vi "Launch Nested Actors.vi"(8 "error in (no error)":errorcluster, 11 "Preparation Line in":refnum<class "Preparation Line.lvclass">) -> (0 "error out":errorcluster, 3 "Preparation Line out":refnum<class "Preparation Line.lvclass">)   [LabVIEW 2015, in "cRIO-Carbondioxide.lvlib" / "CO2-Actor.lvlib" / "Preparation Line.lvclass"]
uses:
  Preparation Line.lvclass
  <vilib>/ActorFramework/Actor/Actor.lvclass
  Valve/Action.ctl
  Preparation Line.lvclass/Preparation Line.ctl
  CO2 Actor/CO2 Actor.lvclass
  Valve/Valve.lvclass
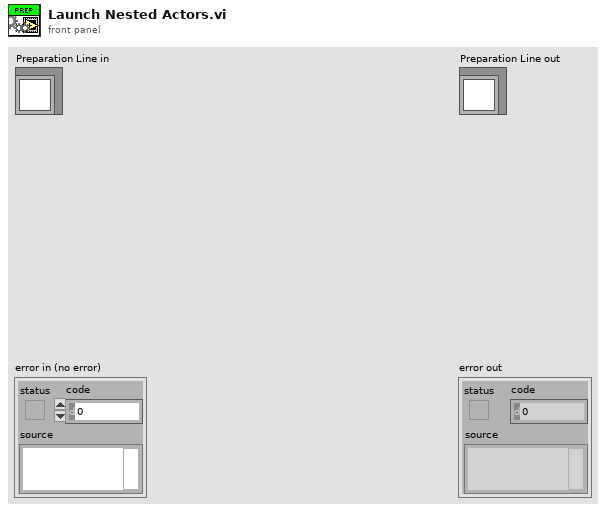
[diagram p1: front panel]
types:
  T1 = typedef "Action.ctl" = enum16{"Open", "Close", "None"}
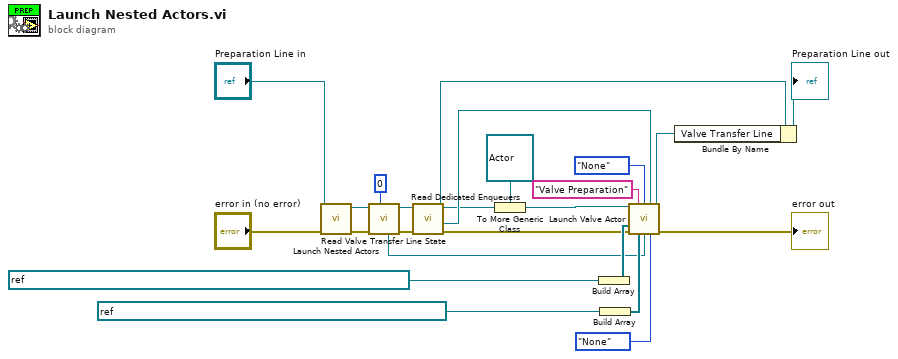
[diagram p0: block diagram]
diagram:
  n1 = call-parent "Launch Nested Actors.vi"("error in (no error)"="error in (no error)", "CO2 Actor in"="Preparation Line in") -> ("error out"=w8:errorcluster, "CO2 Actor out"=w5:refnum<class "Preparation Line.lvclass">)  [unwired: 8 in]
  n2 = call "Read Valve Transfer Line State.vi"("timeout in ms (-1)"=0, "error in (no error)"=w8, "Preparation Line in"=w5) -> ("error out"=w7:errorcluster, "Preparation Line out"=w6:refnum<class "Preparation Line.lvclass">, "Valve Prep Line StateQ"=w3:refnum<queue>)  [unwired: 5 in, 1 out]
  n3 = call "Read Dedicated Enqueuers.vi"("error in (no error)"=w7, "CO2 Actor in"=w6) -> ("error out"=w10:errorcluster, "DedicatedEnQrs"=w9:refnum<queue>, "CO2 Actor out"=w4:refnum<class "Preparation Line.lvclass">)  [unwired: 6 in, 1 out]
  n4 = To More Generic Class(target class=refnum<class "Actor.lvclass"> refnum ("Caller Actor in"), reference=w4) -> (generic class reference=w17:refnum<class "Actor.lvclass">)
  n5 = Build Array(refnum<k21> "ni.var.psp://crio-carbondioxide/AMS Gas SHV/Valves/Prep Line Valve 0" ("SHV")) -> (w11:refnum<k21>[])
  n6 = Build Array(refnum<k21> "ni.var.io://crio-carbondioxide/Mod2/Prep Line Valve 0 DV300" ("SHV")) -> (w19:refnum<k21>[])
  n7 = call "Launch Valve Actor.vi"("Caller Actor in"=w17, "Name"="Valve Preparation", "Start Action (Open)"=Action."None", "DedicatedEnQrs"=w9, "SHV Aliases"=w11, "error in (no error)"=w10, "SHV"=w19, "StateQ"=w3, "Stop Action (Close)"=Action."None") -> ("Caller-To-Actor Enqueuer"=w13:refnum<class "Message Enqueuer.lvclass">, "error out"=→"error out":errorcluster)  [unwired: 5 in]
  n8 = Bundle By Name(cluster=w4, "Valve Transfer Line"=w13) -> (→"Preparation Line out":refnum<class "Preparation Line.lvclass">)
